vi "按灯CTR.vi"(0 "Data In":T3={"设备名称"="", "操作人员"="", "设备状态"=enum."设备缺料", "附加信息"=""} caption="数据输入", 2 "Display State In":T2={"Data"={"设备名称"="", "操作人员"="", "设备状态"=enum."设备缺料", "附加信息"=""}} caption="显示状态输入", 3 "Container State":T4 caption="容器状态") -> (6 "Data Out":T3={"设备名称"="", "操作人员"="", "设备状态"=enum."设备缺料", "附加信息"=""} caption="数据输出", 7 "Display State Out":T2={"Data"={"设备名称"="", "操作人员"="", "设备状态"=enum."设备缺料", "附加信息"=""}} caption="显示状态输出", 8 "Action":T1 caption="动作")   [LabVIEW 2020, in "按灯CTR.xctl"]
uses:
  <vilib>/_xctls/Container State.ctl
  <vilib>/_xctls/Action.ctl
  <vilib>/_xctls/XControlSupport.lvlib
panel:
  out "设备名称":bool
  out "颜色盒 3":u32(colorbox)=9868950
  out "操作员":string
  out "颜色盒 4":u32(colorbox)=9868950
  out "颜色盒 5":u32(colorbox)=9868950
  out "设备状态":string
  out "颜色盒 6":u32(colorbox)=9868950
  in  "上线":bool=TRUE
  out "提示信息":string
  out "颜色盒":u32(colorbox)=9868950
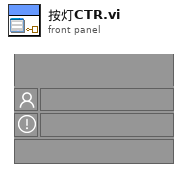
[diagram p1: front panel]
types:
  T1 = typedef "XControlSupport.lvlib/Action.ctl" = cluster{"Data Changed?":bool, "State Changed?":bool, "Action Name":string}
  T2 = typedef "按灯CTR.xctl/按灯CTR状态.ctl" = cluster{"Data":T3}
  T3 = typedef "按灯CTR.xctl/按灯CTR数据.ctl" = cluster{"设备名称":string, "操作人员":string, "设备状态":enum16{"设备离线", "设备正常", "设备缺料", "设备故障", "质量报警"}, "附加信息":string}
  T4 = typedef "XControlSupport.lvlib/Container State.ctl" = cluster{"Indicator?":bool, "Run Mode?":bool, " Refnum":refnum<vi>}
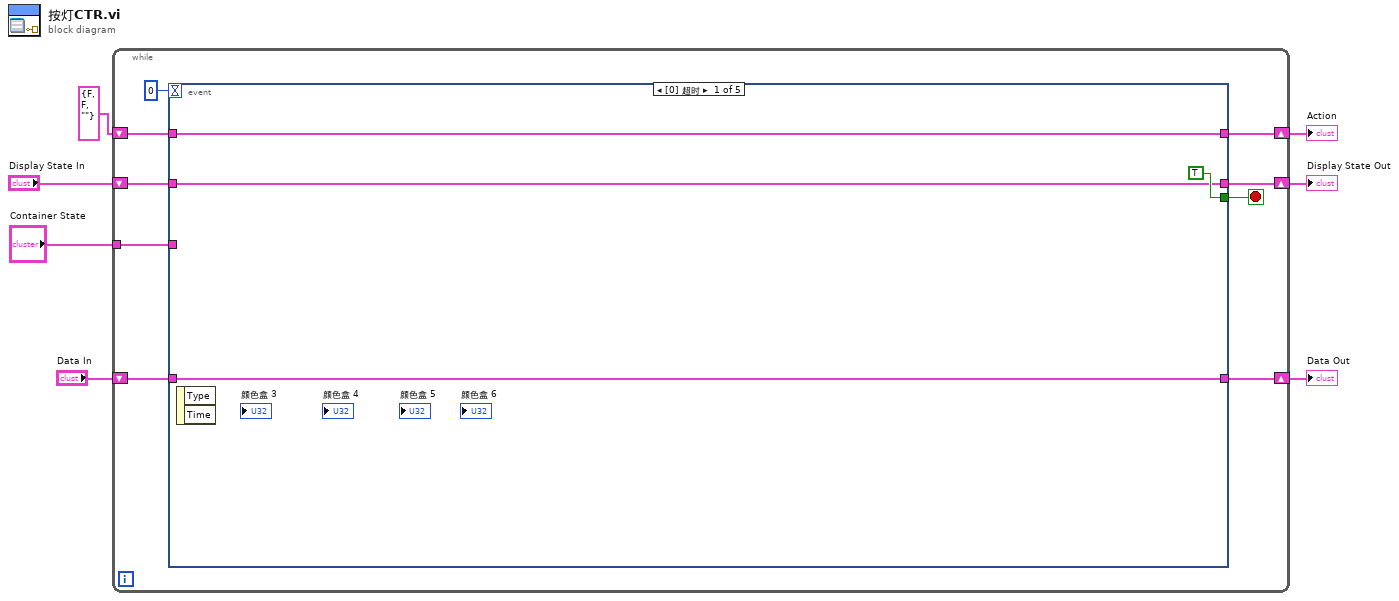
[diagram p0: block diagram]
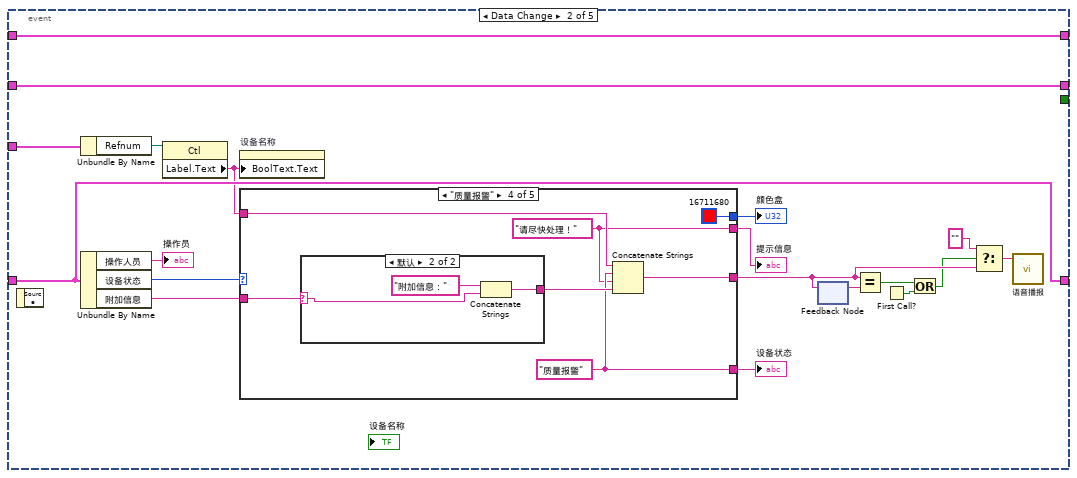
[diagram p2: hidden frame]
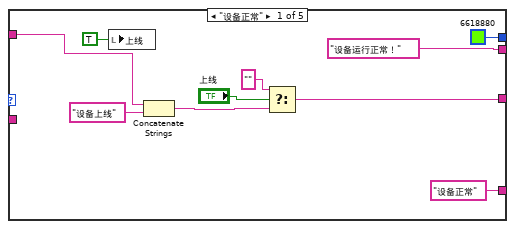
[diagram p3: hidden frame]
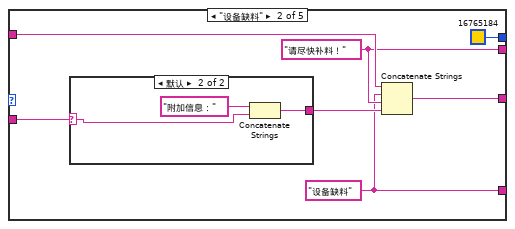
[diagram p4: hidden frame]
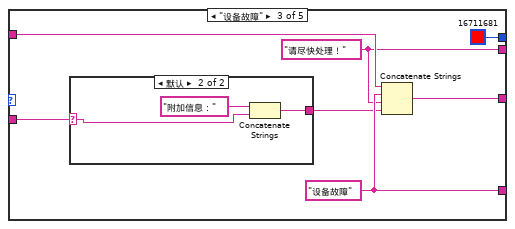
[diagram p6: hidden frame]
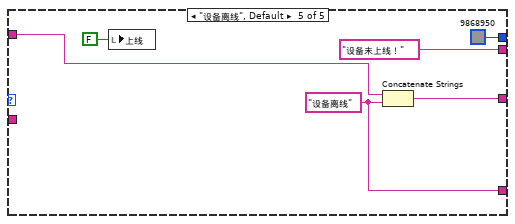
[diagram p9: hidden frame]
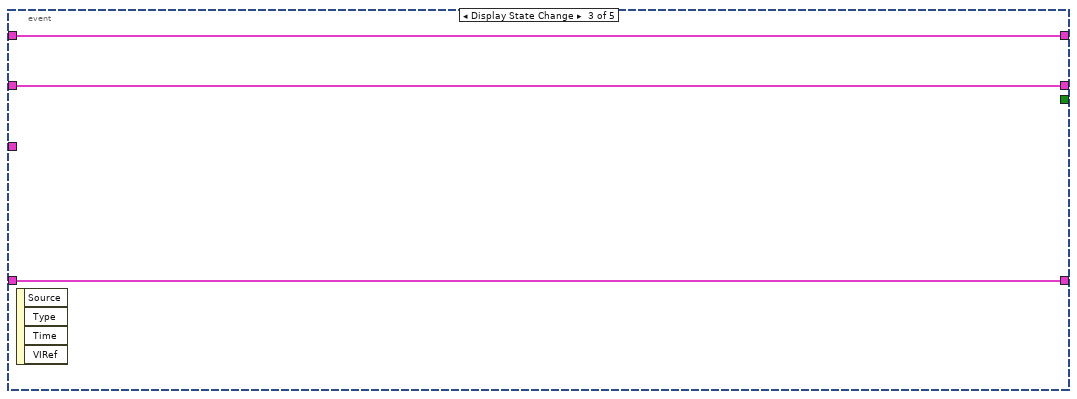
[diagram p10: hidden frame]
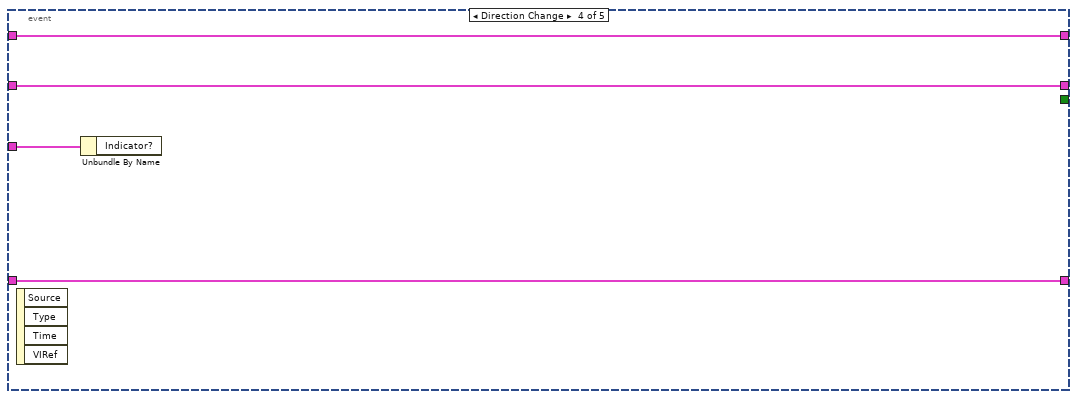
[diagram p11: hidden frame]
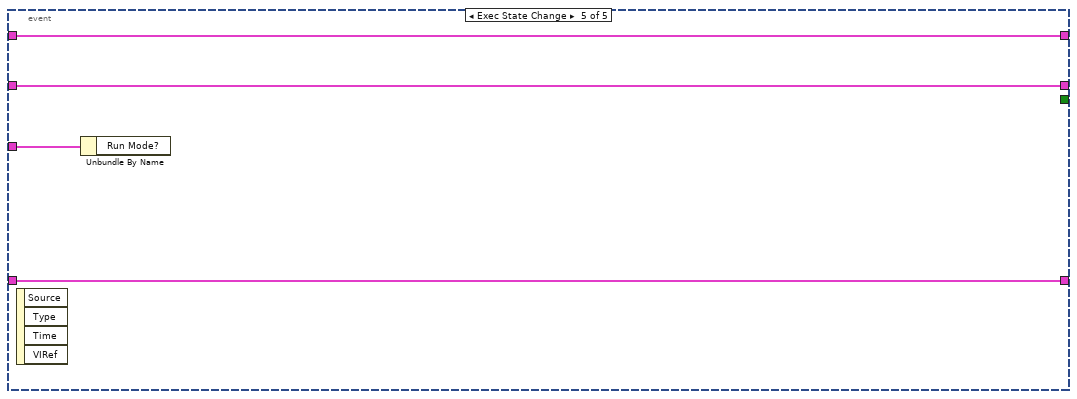
[diagram p12: hidden frame]
diagram:
  n1 = while {
    shift-right: [w15] -> w4
    shift-left: "Display State In" -> [w16]
    tunnel: "Container State" -> [w12]
    shift-right: [w10] -> w7
    shift-left: "Data In" -> [w11]
    shift-right: [w8] -> w2
    shift-left: T1 {"Data Changed?"=FALSE, "State Changed?"=FALSE, "Action Name"=""} ("Action") -> [w9]
    stop <- w14 stop-if-true
    n2 = event shown="[0] 超时" {
      selector: _ -> [_ _ _ _ _]
      dyn-events: _ -> [_ _ _ _ _]
      timeout: 0 -> [_ _ _ _ _]
      tunnel: w16 -> [w18 w31 w88 w91 w95]
      tunnel: [w18 w31 w88 w91 w95] -> w15
      tunnel: [TRUE _ _ _ _] -> w14
      tunnel: w12 -> [_ w30 _ w92 w96]
      tunnel: w11 -> [w17 w33 w87 w90 w94]
      tunnel: [w17 w33 w87 w90 w94] -> w10
      tunnel: [w19 w39 w86 w89 w93] -> w8
      tunnel: w9 -> [w19 w39 w86 w89 w93]
      event Timeout {
        n3 = event-data() -> ()  [unwired: 1 in, 2 out]
      }
      event Data Change {
        n4 = event-data() -> ()  [unwired: 1 in, 1 out]
        n5 = Unbundle By Name(w30) -> ("Refnum"=w29:refnum<vi>)
        n6 = Unbundle By Name(w33) -> ("操作人员"=→"操作员":string, "设备状态"=w36:enum16{"设备离线", "设备正常", "设备缺料", "设备故障", "质量报警"}, "附加信息"=w35:string)
        n7 = property class="Ctl"(reference=w29) -> ("Label.Text"=w21:string)  [unwired: 1 in, 2 out]
        n8 = property on="设备名称" class="Bool (严格)"("BoolText.Text"=w21) -> ()  [unwired: 2 in, 2 out]
        n9 = case shown="\"质量报警\"" w36 {
          tunnel: ["设备运行正常！" ("字符串") w54 w61 w71 "设备未上线！" ("字符串")] -> w38
          tunnel: [u32 6618880 ("颜色盒") u32 16765184 ("颜色盒") u32 16711681 ("颜色盒") u32 16711680 ("颜色盒") u32 9868950 ("颜色盒")] -> w37
          tunnel: w35 -> [_ w52 w65 w70 _]
          tunnel: w21 -> [w45 w55 w64 w73 w84]
          tunnel: [w44 w53 w63 w72 w83] -> w26
          tunnel: ["设备正常" ("字符串") w50 w62 w74 w82] -> w32
          frame "设备正常" {
            n10 = local write "上线"(TRUE ("上线")) -> ()
            n11 = Concatenate Strings(w45, "设备上线" ("字符串")) -> (w42:string)
            n12 = Select(t="", s="上线", f=w42) -> (s? t:f=w44:string)
          }
          frame "设备缺料" {
            w54 = "请尽快补料！" ("字符串")
            w50 = "设备缺料" ("字符串")
            n13 = case shown="默认" w52 {
              selector: w52 -> [_ w57]
              tunnel: [_ w58] -> w51
              frame "" {
              }
              frame Default {
                n14 = Concatenate Strings("附加信息：" ("字符串"), w57) -> (w58:string)
              }
            }
            n15 = Concatenate Strings(w55, w50, w54, w51) -> (w53:string)
          }
          frame "设备故障" {
            w61 = "请尽快处理！" ("字符串")
            w62 = "设备故障" ("字符串")
            n16 = case shown="默认" w65 {
              selector: w65 -> [_ w67]
              tunnel: [_ w68] -> w60
              frame "" {
              }
              frame Default {
                n17 = Concatenate Strings("附加信息：" ("字符串"), w67) -> (w68:string)
              }
            }
            n18 = Concatenate Strings(w64, w62, w61, w60) -> (w63:string)
          }
          frame "质量报警" {
            w71 = "请尽快处理！" ("字符串")
            w74 = "质量报警" ("字符串")
            n19 = case shown="默认" w70 {
              selector: w70 -> [_ w77]
              tunnel: [_ w78] -> w75
              frame "" {
              }
              frame Default {
                n20 = Concatenate Strings("附加信息：" ("字符串"), w77) -> (w78:string)
              }
            }
            n21 = Concatenate Strings(w73, w74, w71, w75) -> (w72:string)
          }
          frame "设备离线", Default {
            w82 = "设备离线" ("字符串")
            n22 = local write "上线"(FALSE ("上线")) -> ()
            n23 = Concatenate Strings(w84, w82) -> (w83:string)
          }
        }
        "提示信息" <- w38
        "颜色盒" <- w37
        "设备状态" <- w32
        n24 = feedback-in #1(w26) -> ()
        n25 = feedback #1() -> (w28:string)  [unwired: 1 in]
        n26 = Equal?(x=w26, y=w28) -> (x = y?=w23:bool)
        n27 = First Call?() -> (First Call?: T/F=w22:bool)
        n28 = Or(x=w23, y=w22) -> (x .or. y?=w24:bool)
        n29 = Select(t="", s=w24, f=w26) -> (s? t:f=w25:string)
        n30 = call "语音播报.vi"("textToSpeak"=w25) -> ()  [unwired: 10 in, 1 out]
      }
      event Display State Change {
        n31 = event-data() -> ()  [unwired: 1 in, 4 out]
      }
      event Direction Change {
        n32 = event-data() -> ()  [unwired: 1 in, 4 out]
        n33 = Unbundle By Name(w92) -> ()  [unwired: 1 out]
      }
      event Exec State Change {
        n34 = event-data() -> ()  [unwired: 1 in, 4 out]
        n35 = Unbundle By Name(w96) -> ()  [unwired: 1 out]
      }
    }
  }
  "Display State Out" <- w4
  "Data Out" <- w7
  "Action" <- w2
